vi "READ.vi"(8 "write buffer":string=":READ?", 11 "VISA resource name":refnum<visa-resource-name>="GPIB0::7::INSTR") -> (0 "error out":errorcluster, 3 "read buffer":string)   [LabVIEW 2016]
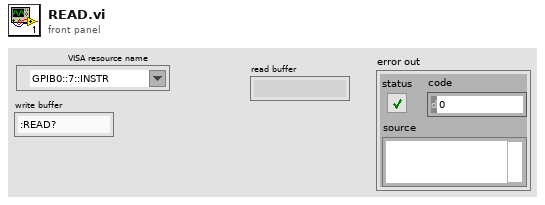
[diagram p1: front panel]
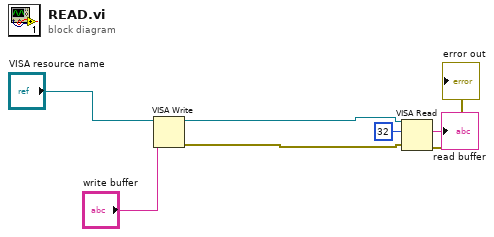
[diagram p0: block diagram]
diagram:
  n1 = VISA Write(VISA resource name="VISA resource name", write buffer="write buffer") -> (VISA resource name out=w4:refnum<visa-resource-name>, error out=w2:errorcluster)  [unwired: 1 in, 1 out]
  n2 = VISA Read(VISA resource name=w4, byte count=u32 32, error in (no error)=w2) -> (read buffer=→"read buffer":string, error out=→"error out":errorcluster)  [unwired: 2 out]
